vi "LoadImage(ImageData).vi"(1 "image data":T1, 5 "error in (no error)":errorcluster) -> (15 "ImageOut":refnum<k24>, 17 "ImageSize":cluster{"Width":i32, "Height":i32}, 19 "error out":errorcluster)   [LabVIEW 2020, in "LcPictureBox.lvclass"]
uses:
  LcPictureBox.lvclass
  System.Drawing
  <vilib>/picture/picture.llb/imagedata.ctl
  <vilib>/wsapi/NI_WebServices.lvlib
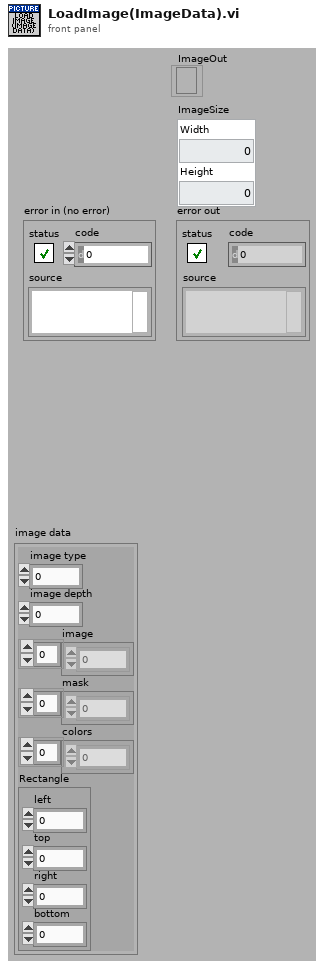
[diagram p1: front panel]
types:
  T1 = typedef "imagedata.ctl" = cluster{"image type":i32, "image depth":i32, "image":u8[], "mask":u8[], "colors":u32[], "Rectangle":cluster{"left":i16, "top":i16, "right":i16, "bottom":i16}}
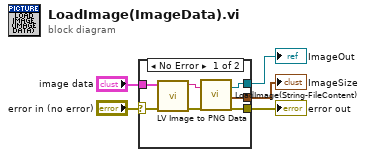
[diagram p0: block diagram]
diagram:
  n1 = case shown="No Error" "error in (no error)" {
    selector: "error in (no error)" -> [w10 w13]
    tunnel: [w8 w13] -> w4
    tunnel: "image data" -> [w12 _]
    tunnel: [w7 _] -> w2
    tunnel: [w6 _] -> w1
    frame No Error {
      n2 = call <vilib>:"LV Image to PNG Data.vi"("error in (no error)"=w10, "image data"=w12) -> ("error out"=w9:errorcluster, "png data"=w11:string)  [unwired: 8 in]
      n3 = call "LoadImage(String-FileContent).vi"("ImageFileContent"=w11, "error in (no error)"=w9) -> ("ImageOut"=w6:refnum<k24>, "ImageSize"=w7:cluster{"Width":i32, "Height":i32}, "error out"=w8:errorcluster)  [unwired: 15 in]
    }
    frame Error {
    }
  }
  "error out" <- w4
  "ImageOut" <- w1
  "ImageSize" <- w2
